vi "Begin.vi"(8 "error in":errorcluster) -> (0 "error out":errorcluster)   [LabVIEW 2019]
doc: "Called before other user functions, this VI is expected to open initial I/O refnums, load in file data, and do all program initialization. Notice that the <B>error out</B> terminal is simply used for data flow. Wiring it to other structures or subVIs ensures that this VI runs first."
uses:
  <vilib>/Rock Robotics/WPI/DriverStation/WPI_DriverStationRobotMode2.ctl
  <vilib>/Rock Robotics/WPI/Joystick/WPI_JoystickDeviceEnum.ctl
  <vilib>/Rock Robotics/SystemInterfaces/DIO/FPGA_DIOChannel.ctl
  <vilib>/Rock Robotics/SystemInterfaces/DIO/FPGA_DIOPWMChannel.ctl
  Robot Global Data.vi
  <vilib>/Rock Robotics/Network Tables/NT Write String Array.vi
  <vilib>/Rock Robotics/WPI/Counter/WPI_CounterDigitalInputToDigitalSource.vi
  <vilib>/Rock Robotics/WPI/RobotDrive/WPI_RobotDriveOpen4MotorWithTalonSRX.vi
  <vilib>/Rock Robotics/WPI/SafetyOutput/WPI_SafetyOutputConfigMenu.ctl
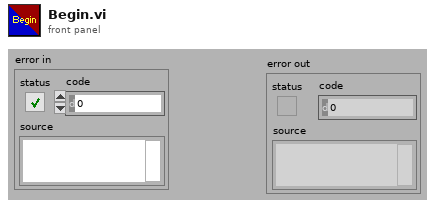
[diagram p1: front panel]
types:
  T1 = typedef "FPGA_DIOPWMChannel.ctl" = enum8{"PWM 0", "PWM 1", "PWM 2", "PWM 3", "PWM 4", "PWM 5", "PWM 6", "PWM 7", "PWM 8", "PWM 9", "PWM MXP 0", "PWM MXP 1", "PWM MXP 2", "PWM MXP 3", "PWM MXP 4", "PWM MXP 5", "PWM MXP 6", "PWM MXP 7", "PWM MXP 8", "PWM MXP 9", "Invalid"}
  T2 = typedef "FPGA_DIOChannel.ctl" = enum8{"DIO 0", "DIO 1", "DIO 2", "DIO 3", "DIO 4", "DIO 5", "DIO 6", "DIO 7", "DIO 8", "DIO 9", "DIO MXP 0", "DIO MXP 1", "DIO MXP 2", "DIO MXP 3", "DIO MXP 4", "DIO MXP 5", "DIO MXP 6", "DIO MXP 7", "DIO MXP 8", "DIO MXP 9", "DIO MXP 10", "DIO MXP 11", "DIO MXP 12", "DIO MXP 13", "DIO MXP 14", "DIO MXP 15", "SPI Port CS1", "SPI Port CS2", "SPI Port CS3", "SPI Port MISO", "SPI Port MOSI", "Invalid"}
  T3 = typedef "WPI_JoystickDeviceEnum.ctl" = enum16{"USB 0", "USB 1", "USB 2", "USB 3", "USB 4", "USB 5"}
  T4 = typedef "WPI_DriverStationRobotMode2.ctl" = enum16{"Autonomous Disabled", "Autonomous Enabled", "Teleop Disabled", "Teleop Enabled", "Disconnected", "Finish", "Test Disabled", "Test Enabled", "Emergency Stopped"}
  T5 = typedef "WPI_SafetyOutputConfigMenu.ctl" = enum16{"Enable", "Disable"}
  T6 = typedef "WPI_RobotDriveDevRef.ctl" = cluster{"DevStatus":errorcluster, "Motors[]":T7[], "Square Inputs":bool, "Max Output":dbl}
  T7 = typedef "WPI_MotorControlDeviceRef.ctl" = cluster{"DeviceStatus":errorcluster, "Type":T8, "PWM":cluster{"PWM Channel":T1, "DeadBand":T9}, "CAN":cluster{"Device Number":u8, "SetOutput VI Ref":variant, "GetOutput VI Ref":variant, "Enable VI Ref":variant, "Disable VI Ref":variant, "Data":variant}, "Invert":bool, "DIO PWM":cluster{"PWM \"Enable\" Channel":T1, "DIOChannel":T2, "PWM Rate":dbl}}
  T8 = typedef "WPI_MotorControlType.ctl" = enum16{"PWM", "CAN", "DIO PWM"}
  T9 = typedef "WPI_PWMDeadband.ctl" = cluster{"Name":string, "maxPositivePwm":i32, "minPositivePwm":i32, "centerPwm":i32, "maxNegativePwm":i32, "minNegativePwm":i32, "angularRange":u16}
  T10 = typedef "WPI_JoystickDevRef.ctl" = cluster{"Device":T3}
  T11 = typedef "WPI_DigitalInputDevRef.ctl" = cluster{"DevStatus":errorcluster, "DIO Channel":T2}
  T12 = typedef "FPGA_CounterEncoderSourceConvertionLVSourceType.ctl" = cluster{"DevStatus":errorcluster, "AnalogTriggerMode?":bool, "DigitalMode":cluster{"DIO Channel":T13}, "AnalogTriggerMode":cluster{"AnalogTriggerIndex":T14, "OutputType":T15}}
  T13 = typedef "FPGA_DIODigitalSourceChannel.ctl" = enum8{"DIO 0", "DIO 1", "DIO 2", "DIO 3", "DIO 4", "DIO 5", "DIO 6", "DIO 7", "DIO 8", "DIO 9", "DIO MXP 0", "DIO MXP 1", "DIO MXP 2", "DIO MXP 3", "DIO MXP 4", "DIO MXP 5", "DIO MXP 6", "DIO MXP 7", "DIO MXP 8", "DIO MXP 9", "DIO MXP 10", "DIO MXP 11", "DIO MXP 12", "DIO MXP 13", "DIO MXP 14", "DIO MXP 15", "SPI Port CS1", "SPI Port CS2", "SPI Port CS3", "SPI Port MISO", "SPI Port MOSI", "Disabled"}
  T14 = typedef "FPGA_AnalogTriggerIndex.ctl" = enum8{"Trig 0", "Trig 1", "Trig 2", "Trig 3", "Trig 4", "Trig 5", "Trig 6", "Trig 7", "Invalid"}
  T15 = typedef "FPGA_AnalogTriggerOutType.ctl" = enum16{"InWindow", "TriggerState", "Rising", "Falling"}
  T16 = typedef "WPI_EncoderDevRef.ctl" = cluster{"DevStatus":errorcluster, "EncoderIndex":T17, "CounterIndex":T18, "DistancePerCount":dbl, "Decoding Type":T19}
  T17 = typedef "FPGA_EncoderIdx.ctl" = enum8{"Enc 0", "Enc 1", "Enc 2", "Enc 3", "Enc 4", "Enc 5", "Enc 6", "Enc 7", "Invalid"}
  T18 = typedef "FPGA_CounterCtrSystemIndex.ctl" = enum8{"Ctr 0", "Ctr 1", "Ctr 2", "Ctr 3", "Ctr 4", "Ctr 5", "Ctr 6", "Ctr 7", "Invalid"}
  T19 = typedef "WPI_EncoderType.ctl" = enum16{"1x", "2x", "4x"}
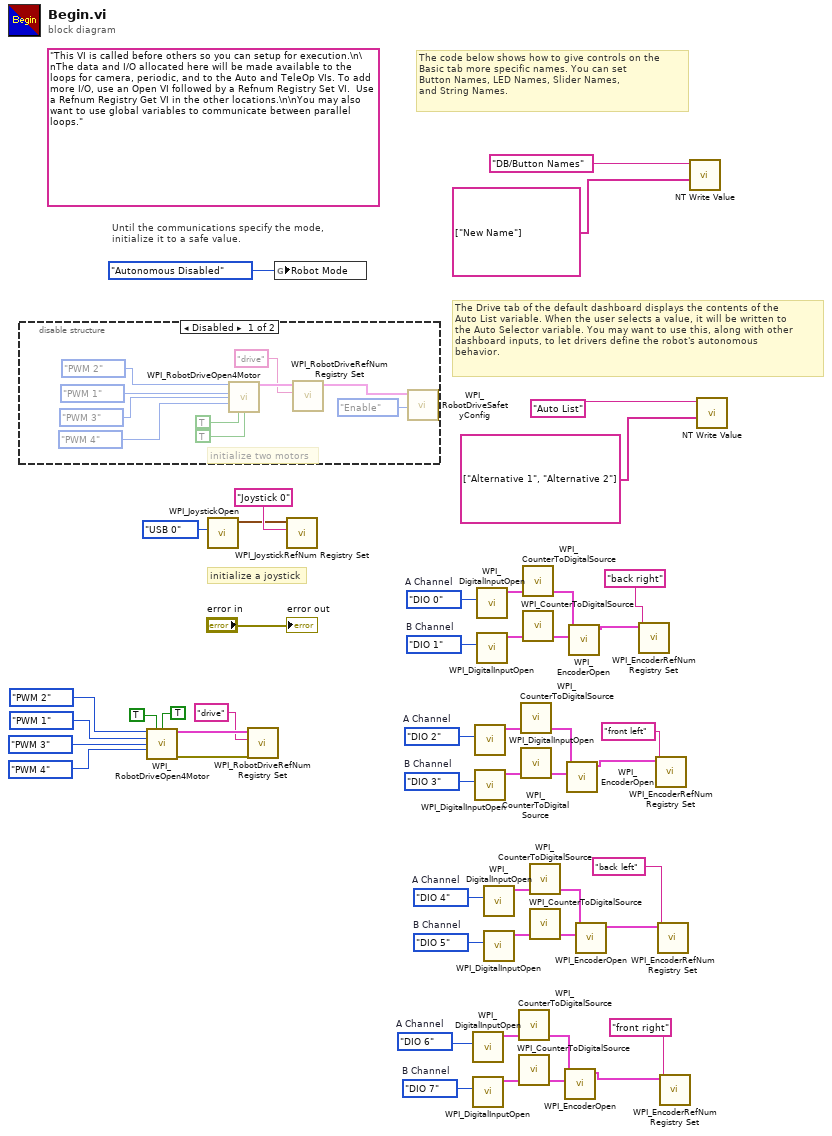
[diagram p0: block diagram]
diagram:
  w23 = FPGA_DIOChannel."DIO 7"  # B Channel
  w22 = FPGA_DIOChannel."DIO 6"  # A Channel
  w29 = FPGA_DIOChannel."DIO 5"  # B Channel
  w28 = FPGA_DIOChannel."DIO 4"  # A Channel
  w35 = FPGA_DIOChannel."DIO 3"  # B Channel
  w34 = FPGA_DIOChannel."DIO 2"  # A Channel
  w41 = FPGA_DIOChannel."DIO 1"  # B Channel
  w40 = FPGA_DIOChannel."DIO 0"  # A Channel
  (unwired) "This VI is called before others so you can setup for execution.\n\nThe data and I/O allocated here will be made available to the loops for camera, periodic, and to the Auto and TeleOp VIs. To add more I/O, use an Open VI followed by a Refnum Registry Set VI.  Use a Refnum Registry Get VI in the other locations.\n\nYou may also want to use global variables to communicate between parallel loops."
  # "The Drive tab of the default dashboard displays the contents of the\nAuto List variable. When the user selects a value, it will be written to\nthe Auto Selector variable. You may want to use this, along with other\ndashboard inputs, to let drivers define the robot's autonomous\nbehavior."
  # "The code below shows how to give controls on the\nBasic tab more specific names. You can set\nButton Names, LED Names, Slider Names,\nand String Names."
  # "initialize a joystick"
  # "Until the communications specify the mode,\ninitialize it to a safe value."
  n1 = disable-structure shown="Disabled" {
    frame Disabled {
      # "initialize two motors"
      n2 = call-poly <vilib>:"WPI_RobotDriveOpen4Motor.vi"("Rear Left Motor"=FPGA_DIOPWMChannel."PWM 2", "Rear Right Motor"=FPGA_DIOPWMChannel."PWM 1", "Front Left Motor"=FPGA_DIOPWMChannel."PWM 3", "Front Right Motor"=FPGA_DIOPWMChannel."PWM 4", "Front Left Motor Inverted"=TRUE, "Front Right Motor Inverted"=TRUE) -> ("RobotDriveDevRef"=w58:T6)  [unwired: 8 in, 1 out]
      n3 = call <vilib>:"WPI_RobotDriveRefNum Registry Set.vi"("refnum name"="drive", "RobotDriveDevRef"=w58) -> ("RobotDriveDevRef"=w60:T6)  [unwired: 2 in, 7 out]
      n4 = call <vilib>:"WPI_RobotDriveSafetyConfig.vi"("mode"=WPI_SafetyOutputConfigMenu."Enable", "RobotDriveDevRef"=w60) -> ()  [unwired: 8 in, 2 out]
    }
    frame Enabled {
    }
  }
  n5 = call-poly <vilib>:"WPI_RobotDriveOpen4Motor.vi"("Rear Left Motor"=FPGA_DIOPWMChannel."PWM 2", "Rear Left Motor Inverted"=TRUE, "Rear Right Motor Inverted"=TRUE, "Rear Right Motor"=FPGA_DIOPWMChannel."PWM 1", "Front Left Motor"=FPGA_DIOPWMChannel."PWM 3", "Front Right Motor"=FPGA_DIOPWMChannel."PWM 4") -> ("RobotDriveDevRef"=w3:T6, "error out"=w2:errorcluster)  [unwired: 8 in]
  n6 = call <vilib>:"WPI_JoystickOpen.vi"("JoystickDevice"=WPI_JoystickDeviceEnum."USB 0") -> ("JoystickDevRef"=w48:T10)  [unwired: 10 in]
  n7 = call <vilib>:"WPI_RobotDriveRefNum Registry Set.vi"("error in (no error)"=w2, "refnum name"="drive", "RobotDriveDevRef"=w3) -> ()  [unwired: 7 in, 2 out]
  n8 = global write "Robot Global Data.vi" "Robot Mode"(WPI_DriverStationRobotMode2."Autonomous Disabled" ("Robot Mode")) -> ()
  n9 = call <vilib>:"WPI_JoystickRefNum Registry Set.vi"("refnum name"="Joystick 0", "JoystickDevRef"=w48) -> ()  [unwired: 8 in, 2 out]
  n10 = call <vilib>:"WPI_DigitalInputOpen.vi"("DIO Channel"=w22) -> ("DigitalInputDevRef"=w19:T11)  [unwired: 1 in, 9 out]
  n11 = call <vilib>:"WPI_DigitalInputOpen.vi"("DIO Channel"=w23) -> ("DigitalInputDevRef"=w20:T11)  [unwired: 1 in, 9 out]
  n12 = call <vilib>:"WPI_DigitalInputOpen.vi"("DIO Channel"=w34) -> ("DigitalInputDevRef"=w31:T11)  [unwired: 1 in, 9 out]
  n13 = call <vilib>:"WPI_DigitalInputOpen.vi"("DIO Channel"=w35) -> ("DigitalInputDevRef"=w32:T11)  [unwired: 1 in, 9 out]
  n14 = call <vilib>:"WPI_DigitalInputOpen.vi"("DIO Channel"=w40) -> ("DigitalInputDevRef"=w37:T11)  [unwired: 1 in, 9 out]
  n15 = call <vilib>:"WPI_DigitalInputOpen.vi"("DIO Channel"=w41) -> ("DigitalInputDevRef"=w38:T11)  [unwired: 1 in, 9 out]
  n16 = call <vilib>:"WPI_DigitalInputOpen.vi"("DIO Channel"=w28) -> ("DigitalInputDevRef"=w25:T11)  [unwired: 1 in, 9 out]
  n17 = call <vilib>:"WPI_DigitalInputOpen.vi"("DIO Channel"=w29) -> ("DigitalInputDevRef"=w26:T11)  [unwired: 1 in, 9 out]
  n18 = call-poly <vilib>:"WPI_CounterToDigitalSource.vi"("DigitalInputDevRef"=w19) -> ("Digital Source"=w18:T12)  [unwired: 6 out]
  n19 = call-poly <vilib>:"WPI_CounterToDigitalSource.vi"("DigitalInputDevRef"=w20) -> ("Digital Source"=w21:T12)  [unwired: 6 out]
  n20 = call-poly <vilib>:"WPI_CounterToDigitalSource.vi"("DigitalInputDevRef"=w31) -> ("Digital Source"=w30:T12)  [unwired: 6 out]
  n21 = call-poly <vilib>:"WPI_CounterToDigitalSource.vi"("DigitalInputDevRef"=w32) -> ("Digital Source"=w33:T12)  [unwired: 6 out]
  n22 = call-poly <vilib>:"WPI_CounterToDigitalSource.vi"("DigitalInputDevRef"=w37) -> ("Digital Source"=w36:T12)  [unwired: 6 out]
  n23 = call-poly <vilib>:"WPI_CounterToDigitalSource.vi"("DigitalInputDevRef"=w38) -> ("Digital Source"=w39:T12)  [unwired: 6 out]
  n24 = call-poly <vilib>:"WPI_CounterToDigitalSource.vi"("DigitalInputDevRef"=w25) -> ("Digital Source"=w24:T12)  [unwired: 6 out]
  n25 = call-poly <vilib>:"WPI_CounterToDigitalSource.vi"("DigitalInputDevRef"=w26) -> ("Digital Source"=w27:T12)  [unwired: 6 out]
  n26 = call <vilib>:"WPI_EncoderOpen.vi"("BSource"=w21, "ASource"=w18) -> ("EncoderDevRef"=w12:T16)  [unwired: 6 in, 3 out]
  n27 = call <vilib>:"WPI_EncoderOpen.vi"("BSource"=w33, "ASource"=w30) -> ("EncoderDevRef"=w16:T16)  [unwired: 6 in, 3 out]
  n28 = call <vilib>:"WPI_EncoderOpen.vi"("BSource"=w39, "ASource"=w36) -> ("EncoderDevRef"=w17:T16)  [unwired: 6 in, 3 out]
  n29 = call <vilib>:"WPI_EncoderOpen.vi"("BSource"=w27, "ASource"=w24) -> ("EncoderDevRef"=w14:T16)  [unwired: 6 in, 3 out]
  n30 = call <vilib>:"WPI_EncoderRefNum Registry Set.vi"("refnum name"="back right", "EncoderDevRef"=w17) -> ()  [unwired: 8 in, 2 out]
  n31 = call <vilib>:"WPI_EncoderRefNum Registry Set.vi"("refnum name"="front left", "EncoderDevRef"=w16) -> ()  [unwired: 8 in, 2 out]
  n32 = call <vilib>:"WPI_EncoderRefNum Registry Set.vi"("refnum name"="back left", "EncoderDevRef"=w14) -> ()  [unwired: 8 in, 2 out]
  n33 = call <vilib>:"WPI_EncoderRefNum Registry Set.vi"("refnum name"="front right", "EncoderDevRef"=w12) -> ()  [unwired: 8 in, 2 out]
  n34 = call-poly <vilib>:"NT Write Value.vi"("String Array"=string[] ["New Name"], "Name"="DB/Button Names") -> ()  [unwired: 9 in, 1 out]
  n35 = call-poly <vilib>:"NT Write Value.vi"("String Array"=string[] ["Alternative 1", "Alternative 2"], "Name"="Auto List") -> ()  [unwired: 9 in, 1 out]
  "error out" <- "error in"
